vi "gcz1.vi"(8 "C(k-1)":dbl, 9 "e(k-2)":dbl, 10 "e(k-1)":dbl, 11 "e(k)":dbl) -> (2 "C(k)":dbl)   [LabVIEW 2019]
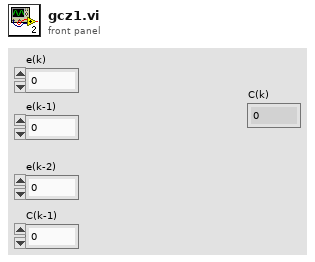
[diagram p1: front panel]
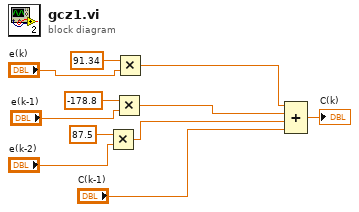
[diagram p0: block diagram]
diagram:
  n1 = Multiply(x=87.5, y="e(k-2)") -> (x*y=w4:dbl)
  n2 = Multiply(x=-178.8, y="e(k-1)") -> (x*y=w5:dbl)
  n3 = Multiply(x=91.34, y="e(k)") -> (x*y=w6:dbl)
  n4 = Compound Arithmetic op=ADD(w6, w5, w4, "C(k-1)") -> (→"C(k)":dbl)
